vi "PWM_PanelSim_Global.vi"(0 "menu":T4=enum."get", 5 "PWMChannel":T3, 7 "Boolean Value":bool, 9 "Numeric Value":dbl format="%#.4f", 11 "error in (no error)":errorcluster, 12 "String Value":string) -> (10 "Value get":T1, 15 "error out":errorcluster)   [LabVIEW 2019]
doc: "This is used to set and get the last motor output values. This is needed for simulation, since we cannot read these values from the hardware.\n\nThis software is licensed. Open the labview\\readme\\WPI Robotics Library Open Source License.txt file for more information."
uses:
  PWM data proto.ctl
  PWM proto.ctl
  PWM Update Ops.ctl
  <vilib>/Rock Robotics/SystemInterfaces/DIO/FPGA_DIOPWMChannel.ctl
panel:
  out "All Values":T1[](array[typedef])
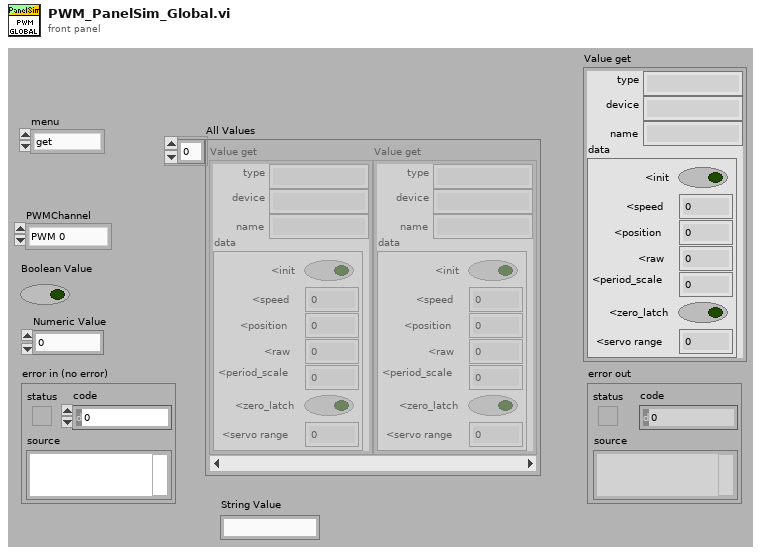
[diagram p1: front panel]
types:
  T1 = typedef "PWM proto.ctl" = cluster{"type":string, "device":string, "name":string, "data":T2}
  T2 = typedef "PWM data proto.ctl" = cluster{"<init":bool, "<speed":dbl, "<position":dbl, "<raw":dbl, "<period_scale":dbl, "<zero_latch":bool, "<servo range":dbl}
  T3 = typedef "FPGA_DIOPWMChannel.ctl" = enum8{"PWM 0", "PWM 1", "PWM 2", "PWM 3", "PWM 4", "PWM 5", "PWM 6", "PWM 7", "PWM 8", "PWM 9", "PWM MXP 0", "PWM MXP 1", "PWM MXP 2", "PWM MXP 3", "PWM MXP 4", "PWM MXP 5", "PWM MXP 6", "PWM MXP 7", "PWM MXP 8", "PWM MXP 9", "Invalid"}
  T4 = typedef "PWM Update Ops.ctl" = enum16{"set init", "set speed", "set position", "set raw", "set  period_scale", "set zero_latch", "set angular range", "get", "delete", "JSON update", "set name", "transmit initial", "reset"}
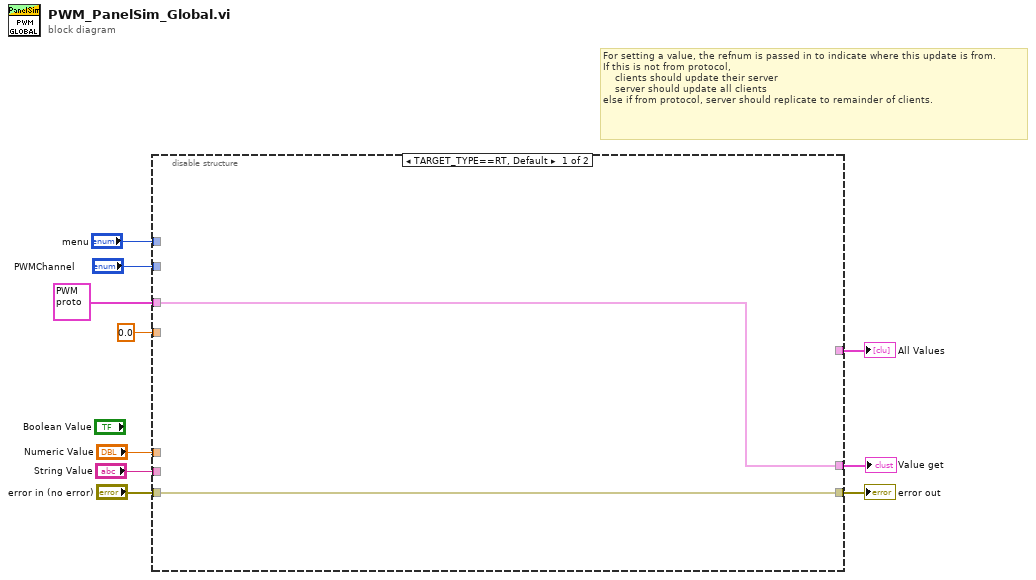
[diagram p0: block diagram]
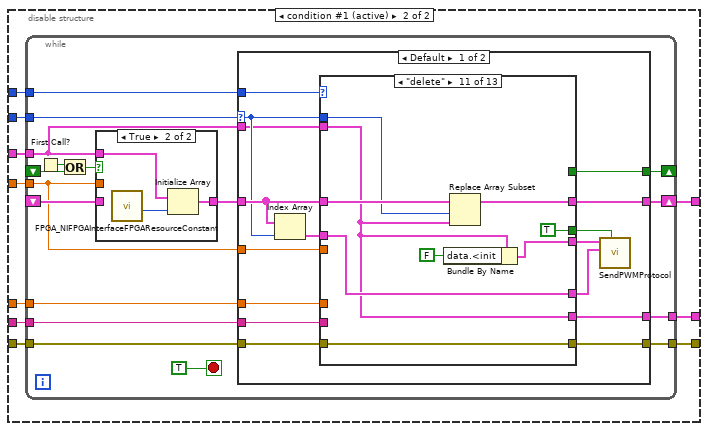
[diagram p2: hidden frame]
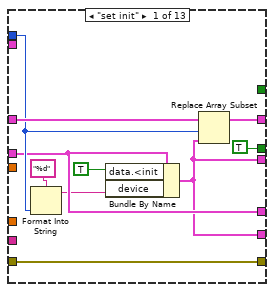
[diagram p3: hidden frame]
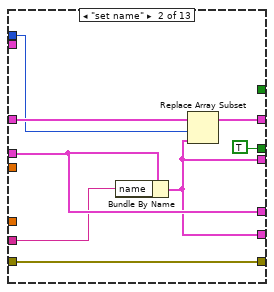
[diagram p4: hidden frame]
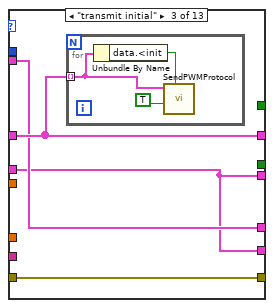
[diagram p5: hidden frame]
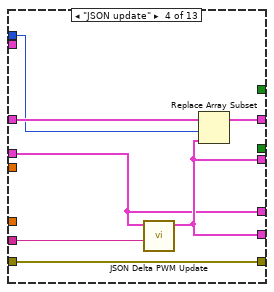
[diagram p6: hidden frame]
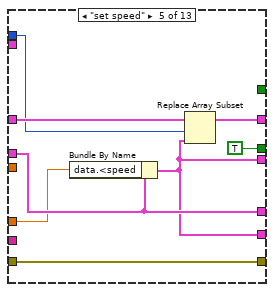
[diagram p7: hidden frame]
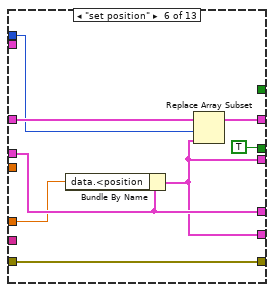
[diagram p8: hidden frame]
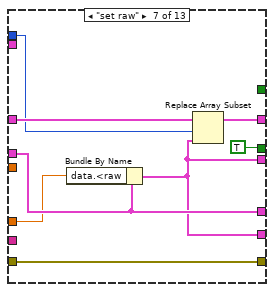
[diagram p9: hidden frame]
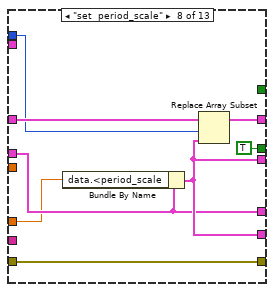
[diagram p10: hidden frame]
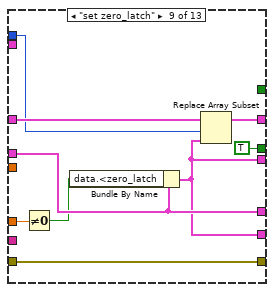
[diagram p11: hidden frame]
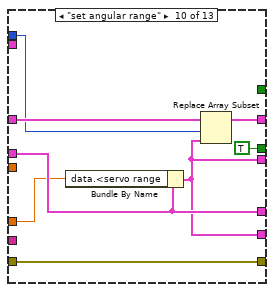
[diagram p12: hidden frame]
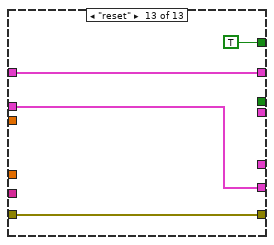
[diagram p14: hidden frame]
diagram:
  # "For setting a value, the refnum is passed in to indicate where this update is from.\nIf this is not from protocol,\n    clients should update their server\n    server should update all clients\nelse if from protocol, server should replicate to remainder of clients."
  n1 = disable-structure shown="TARGET_TYPE==RT, Default" {
    disable-tunnel: "menu" -> [_ w22]
    disable-tunnel: [w12 w21] -> w9
    disable-tunnel: "error in (no error)" -> [w12 w20]
    disable-tunnel: [_ w19] -> w7
    disable-tunnel: 0.0 ("Output") -> [_ w18]
    disable-tunnel: "Numeric Value" -> [_ w17]
    disable-tunnel: "PWMChannel" -> [_ w16]
    disable-tunnel: [w11 w15] -> w3
    disable-tunnel: T1 {"type"="PWM", "device"="", "name"="", "data"={"<init"=FALSE, "<speed"=0.0, "<position"=0.0, "<raw"=0.0, "<period_scale"=0.0, "<zero_latch"=FALSE, "<servo range"=0.0}} -> [w11 w14]
    disable-tunnel: "String Value" -> [_ w13]
    frame condition #0 {
    }
    frame condition #1 (active) {
      n2 = while {
        tunnel: w17 -> [w39]
        tunnel: w20 -> [w35]
        shift-right: [w38] -> w19
        shift-left: _ -> [w31]
        tunnel: [w37] -> w15
        tunnel: w22 -> [w36]
        tunnel: [w34] -> w21
        tunnel: w16 -> [w29]
        tunnel: w18 -> [w30]
        tunnel: w14 -> [w28]
        tunnel: w13 -> [w27]
        shift-right: [w23] -> _
        shift-left: _ -> [w24]
        stop <- TRUE stop-if-true
        n3 = First Call?() -> (First Call?: T/F=w26:bool)
        n4 = Or(x=w26, y=w24) -> (x .or. y?=w25:bool)
        n5 = case shown="True" w25 {
          tunnel: [w156 w159] -> w32
          tunnel: w31 -> [w156 _]
          tunnel: w30 -> [_ _]
          tunnel: w28 -> [_ w157]
          frame False {
          }
          frame True {
            n6 = call <vilib>:"FPGA_NIFPGAInterfaceFPGAResourceConstant.vi"() -> ("NumberOfPWMs"=w158:u32)  [unwired: 11 out]
            n7 = Initialize Array(w157, w158) -> (w159:T1[])
          }
        }
        n8 = case shown="Default" w29 {
          selector: w29 -> [w47 _]
          tunnel: w39 -> [w55 _]
          tunnel: [w54 w155] -> w38
          tunnel: [w53 w153] -> w37
          tunnel: w36 -> [w52 _]
          tunnel: w35 -> [w51 w154]
          tunnel: [w50 w154] -> w34
          tunnel: w32 -> [w49 w155]
          tunnel: w30 -> [w48 _]
          tunnel: w28 -> [w42 w153]
          tunnel: w27 -> [w41 _]
          tunnel: [w40 _] -> w23
          frame Default {
            n9 = Index Array(array=w49, index=w47) -> (element=w46:T1)
            n10 = case shown="\"delete\"" w52 {
              tunnel: w55 -> [_ _ _ _ w89 w96 w104 w112 w123 w129 _ _ _]
              tunnel: [w65 w73 w76 w87 w95 w103 w111 w119 w128 w136 w144 w148 w152] -> w54
              tunnel: w49 -> [w63 w71 w76 w85 w93 w101 w109 w117 w126 w134 w145 w148 w152]
              tunnel: [w56 w67 w74 w83 w88 w97 w105 w114 w121 w130 w138 w146 w150] -> w53
              tunnel: [w64 w72 w77 w86 w94 w102 w110 w118 w127 w135 w143 w147 w151] -> w50
              tunnel: w51 -> [w64 w72 w77 w86 w94 w102 w110 w118 w127 w135 w143 w147 w151]
              tunnel: w47 -> [w60 w69 _ w84 w91 w99 w107 w115 w124 w132 w140 _ _]
              tunnel: w48 -> [_ _ _ _ _ _ _ _ _ _ _ _ _]
              tunnel: [w56 w67 w74 w83 w88 w97 w105 w114 w121 w130 w139 _ _] -> w44
              tunnel: [w59 w68 w75 w82 w90 w98 w106 w113 w122 w131 w141 _ _] -> w43
              tunnel: [TRUE TRUE _ _ TRUE TRUE TRUE TRUE TRUE TRUE TRUE _ _] -> w45
              tunnel: w46 -> [w59 w68 w74 w82 w90 w98 w106 w113 w122 w131 w141 w146 w150]
              tunnel: w42 -> [_ _ w75 _ _ _ _ _ _ _ w138 _ _]
              tunnel: w41 -> [_ w66 _ w81 _ _ _ _ _ _ _ _ _]
              tunnel: [_ _ _ _ _ _ _ _ _ _ _ _ TRUE] -> w40
              frame "set init" {
                n11 = Format Into String(format string="%d", w60) -> (resulting string=w57:string)  [unwired: 2 in, 1 out]
                n12 = Bundle By Name(cluster=w59, "data.<init"=TRUE, "device"=w57) -> (w56:T1)
                n13 = Replace Array Subset(array=w63, new element=w56, index=w60) -> (w65:T1[])
              }
              frame "set name" {
                n14 = Bundle By Name(cluster=w68, "name"=w66) -> (w67:T1)
                n15 = Replace Array Subset(array=w71, new element=w67, index=w69) -> (w73:T1[])
              }
              frame "transmit initial" {
                n16 = for {
                  tunnel: w76 -> [w78] mode=indexing
                  n17 = Unbundle By Name(w78) -> ("data.<init"=w80:bool)
                  n18 = call "SendPWMProtocol.vi"("Send"=w80, "Initialize"=TRUE, "new"=w78) -> ()  [unwired: 9 in]
                }
              }
              frame "JSON update" {
                n19 = call "JSON Delta PWM Update.vi"("Delta JSON"=w81, "input"=w82) -> ("output"=w83:T1)  [unwired: 8 in, 1 out]
                n20 = Replace Array Subset(array=w85, new element=w83, index=w84) -> (w87:T1[])
              }
              frame "set speed" {
                n21 = Bundle By Name(cluster=w90, "data.<speed"=w89) -> (w88:T1)
                n22 = Replace Array Subset(array=w93, new element=w88, index=w91) -> (w95:T1[])
              }
              frame "set position" {
                n23 = Bundle By Name(cluster=w98, "data.<position"=w96) -> (w97:T1)
                n24 = Replace Array Subset(array=w101, new element=w97, index=w99) -> (w103:T1[])
              }
              frame "set raw" {
                n25 = Bundle By Name(cluster=w106, "data.<raw"=w104) -> (w105:T1)
                n26 = Replace Array Subset(array=w109, new element=w105, index=w107) -> (w111:T1[])
              }
              frame "set  period_scale" {
                n27 = Bundle By Name(cluster=w113, "data.<period_scale"=w112) -> (w114:T1)
                n28 = Replace Array Subset(array=w117, new element=w114, index=w115) -> (w119:T1[])
              }
              frame "set zero_latch" {
                n29 = Not Equal To 0?(x=w123) -> (x != 0?=w120:bool)
                n30 = Bundle By Name(cluster=w122, "data.<zero_latch"=w120) -> (w121:T1)
                n31 = Replace Array Subset(array=w126, new element=w121, index=w124) -> (w128:T1[])
              }
              frame "set angular range" {
                n32 = Bundle By Name(cluster=w131, "data.<servo range"=w129) -> (w130:T1)
                n33 = Replace Array Subset(array=w134, new element=w130, index=w132) -> (w136:T1[])
              }
              frame "delete" {
                n34 = Bundle By Name(cluster=w138, "data.<init"=FALSE) -> (w139:T1)
                n35 = Replace Array Subset(array=w145, new element=w138, index=w140) -> (w144:T1[])
              }
              frame "get" {
              }
              frame "reset" {
              }
            }
            n36 = call "SendPWMProtocol.vi"("Send"=w45, "old"=w43, "new"=w44) -> ()  [unwired: 9 in]
          }
          frame "Invalid" {
            # "Do nothing if \nchannel is Invalid."
          }
        }
      }
    }
  }
  "error out" <- w9
  "All Values" <- w7
  "Value get" <- w3
